vi "Simple UDP - Receiver.vi"() -> ()   [LabVIEW 2020]
doc: "UDP协议与TCP的区别在于UDP不包括发送数据包信息的错误检查，因此无法保证接收端是否已接收所发数据。\n\nUDP可用于“广播”数据至整个网络，只需指定可包括全部的IP地址(255.255.255.255)以便发送信息至整个网络。 由于路由器或其他网络硬件通常拒绝转发超过一定点的数据，在实际应用中广播范围可能存在限制。"
panel:
  out "状态显示":string
  in  "停止采集 2":bool
  in  "数据采集卡地址 2":string
  # "概述：演示使用UDP函数通过UDP连接接收数据。\n操作步骤：\n1.确保已运行Simple UDP - Sender.vi。\n2.运行VI。\n3.单击停止按钮停止VI。"
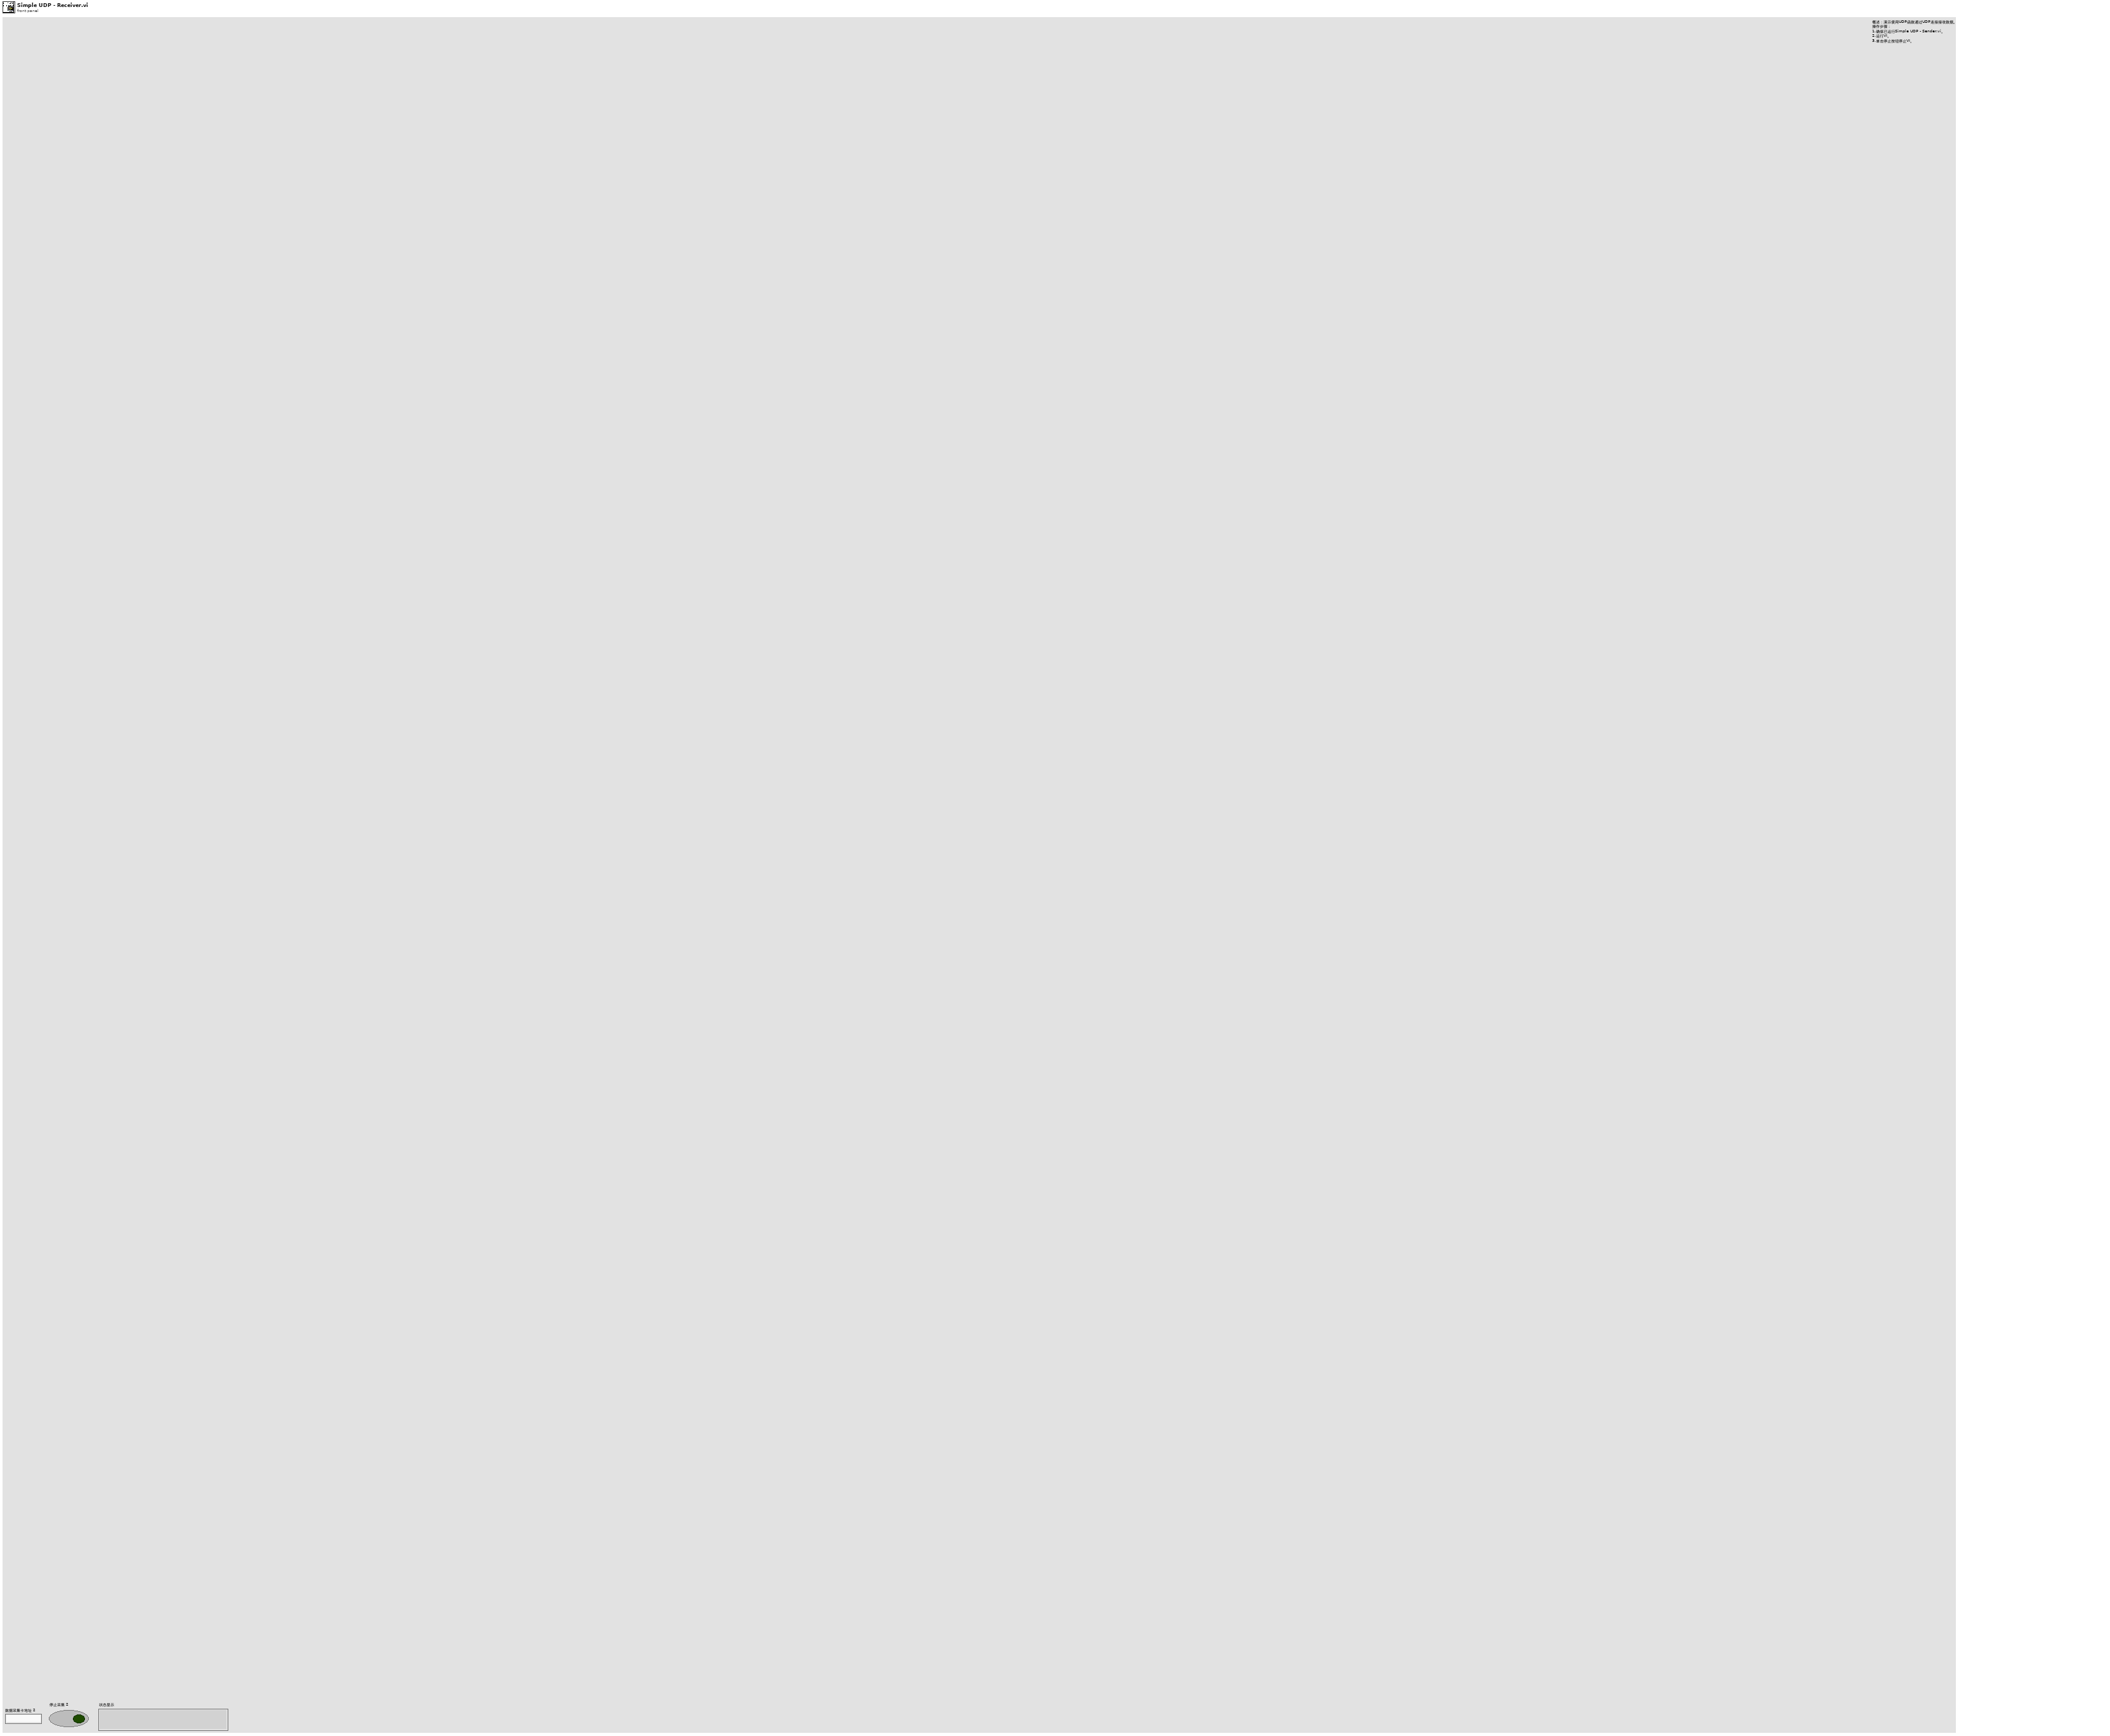
[diagram p1: front panel]
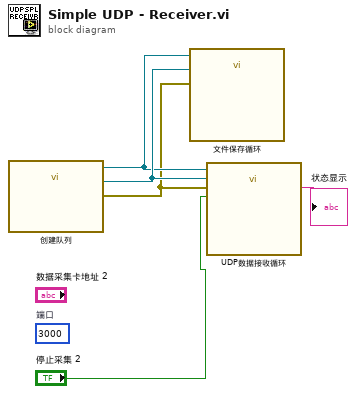
[diagram p0: block diagram]
diagram:
  (unwired) u16 3000  # 端口
  n1 = call "创建队列.vi"() -> ("错误输出"=w3:errorcluster, "结束位队列"=w5:refnum<queue>, "数据队列"=w4:refnum<queue>)  [unwired: 9 in]
  n2 = call "文件保存循环.vi"("错误输入（无错误）"=w3, "结束位队列"=w5, "队列输入"=w4) -> ()  [unwired: 8 in, 1 out]
  n3 = call "UDP数据接收循环.vi"("停止采集"="停止采集 2", "错误输入（无错误）"=w3, "结束位队列"=w5, "队列输入"=w4) -> ("状态显示"=→"状态显示":string)  [unwired: 7 in]
